vi "Init Replies Lists.vi"(8 "error in (no error)":errorcluster, 11 "Monkey in":refnum<class "Tamer.lvclass">) -> (0 "error out":errorcluster, 3 "Monkey out":refnum<class "Tamer.lvclass">)   [LabVIEW 2020, in "Tamer.lvlib" / "Tamer.lvclass"]
uses:
  Tamer.lvclass
  Reply.ctl
  Tamer.lvclass/Tamer.ctl
  a1215997-1aee-4003-9d61-c968e69c494f.vi
  TALOS/TALOS_PPL.lvlibp/Support VIs/Global Constants.vi
  <vilib>/Comparison/Equal/Equal Functor/Equal Functor.lvclass
  TALOS/TALOS_PPL.lvlibp
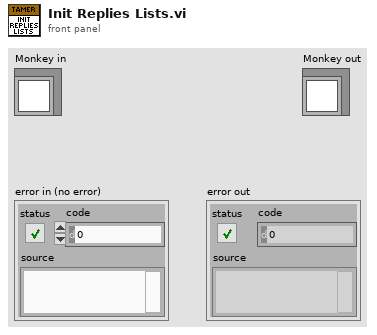
[diagram p1: front panel]
types:
  T1 = typedef "Tamer.lvlib/Tamer.lvclass/Reply.ctl" = cluster{"ID":string, "Status":bool, "GUID":string}
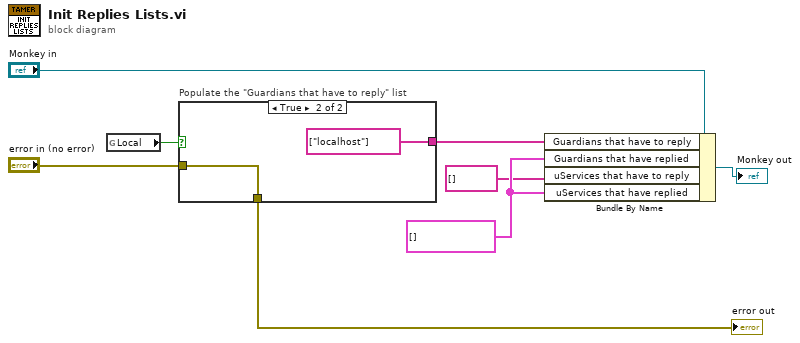
[diagram p0: block diagram]
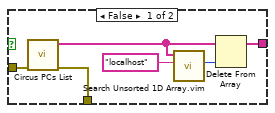
[diagram p2: hidden frame]
diagram:
  w6 = T1[] [] ("uServices that have replied")
  n1 = global read "Global Constants.vi" "Local"() -> (w5:bool)
  n2 = case "Populate the \"Guardians that have to reply\" list" shown="True" w5 {
    tunnel: [w10 string[] ["localhost"] ("Guardians that have to reply")] -> w1
    tunnel: [w14 w16] -> w7
    tunnel: "error in (no error)" -> [w13 w16]
    frame False {
      n3 = call "Circus PCs List.vi"("error in (no error)"=w13) -> ("error out"=w14:errorcluster, "PC List out"=w11:string[])  [unwired: 9 in]
      n4 = call "Search Unsorted 1D Array.vim"("element"="localhost" ("SV Name"), "unsorted 1D array"=w11) -> ("index of element"=w9:i32)  [unwired: 9 in]
      n5 = Delete From Array(array=w11, index=w9) -> (array with subset deleted=w10:string[])  [unwired: 1 in, 1 out]
    }
    frame True {
    }
  }
  "error out" <- w7
  n6 = Bundle By Name(cluster="Monkey in", "Guardians that have to reply"=w1, "Guardians that have replied"=w6, "uServices that have to reply"=string[] [], "uServices that have replied"=w6) -> (→"Monkey out":refnum<class "Tamer.lvclass">)
